vi "Configure Tracking Generator.vi"(6 "Enable Output (F: Disable)":bool, 7 "Output Amplitude (-20 dBm)":dbl=-20.0, 8 "error in (no error)":errorcluster, 9 "Amplitude Step (0 dB)":dbl, 10 "Amplitude Offset (0)":dbl, 11 "VISA resource name":refnum<visa-resource-name>) -> (0 "error out":errorcluster, 3 "VISA resource name out":refnum<visa-resource-name>)   [LabVIEW 2022 SP3, in "Agilent N934X Series.lvlib"]
doc: "Configures the signal characteristics of the tracking generator."
uses:
  <instrlib>/Agilent N934X Series/Agilent N934X Series.lvlib
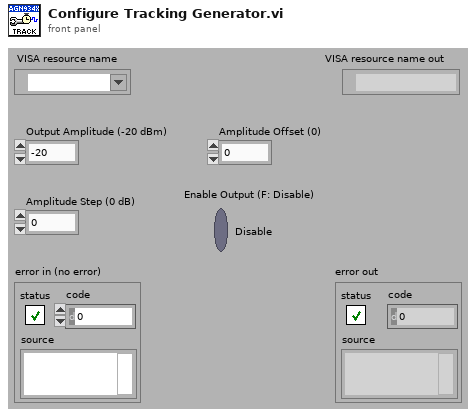
[diagram p1: front panel]
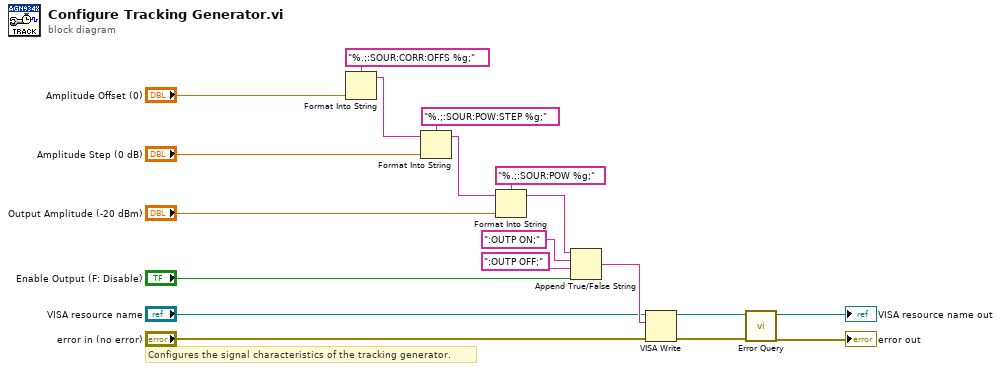
[diagram p0: block diagram]
diagram:
  # "Configures the signal characteristics of the tracking generator."
  n1 = Format Into String(format string="%.;:SOUR:CORR:OFFS %g;", "Amplitude Offset (0)") -> (resulting string=w17:string)  [unwired: 2 in, 1 out]
  n2 = Format Into String(format string="%.;:SOUR:POW:STEP %g;", initial string=w17, "Amplitude Step (0 dB)") -> (resulting string=w14:string)  [unwired: 1 in, 1 out]
  n3 = Format Into String(format string="%.;:SOUR:POW %g;", initial string=w14, "Output Amplitude (-20 dBm)") -> (resulting string=w11:string)  [unwired: 1 in, 1 out]
  n4 = Append True/False String(1:"Enable Output (F: Disable)", 2:":OUTP OFF;", 3:":OUTP ON;", 4:w11) -> (0:w8:string)
  n5 = VISA Write(VISA resource name="VISA resource name", write buffer=w8, error in (no error)="error in (no error)") -> (VISA resource name out=w5:refnum<visa-resource-name>, error out=w4:errorcluster)  [unwired: 1 out]
  n6 = call <instrlib>:"Error Query.vi"("error in (no error)"=w4, "VISA resource name"=w5) -> ("error out"=→"error out":errorcluster, "VISA resource name out"=→"VISA resource name out":refnum<visa-resource-name>)  [unwired: 6 in, 2 out]
